vi "GetGraphVIName.vi"(8 "ErrIn (NoErr)":errorcluster caption="entrée d'erreur (pas d'erreur)", 10 "Curve Index":i32, 11 "Interface In":refnum<class "Interface.lvclass"> caption="DNL_LabVIEW Object in") -> (0 "error out":errorcluster caption="sortie d'erreur", 1 "GraphIndex":i32, 2 "GraphViNames":string[](array[string]), 3 "Interface Out":refnum<class "Interface.lvclass"> caption="DNL_LabVIEW Object out", 4 "GraphCount":i32, 6 "GraphNumbers":i32[](array[numeric]))   [LabVIEW 2019, in "Interface.lvclass"]
uses:
  Interface.lvclass
  Interface.lvclass/Interface.ctl
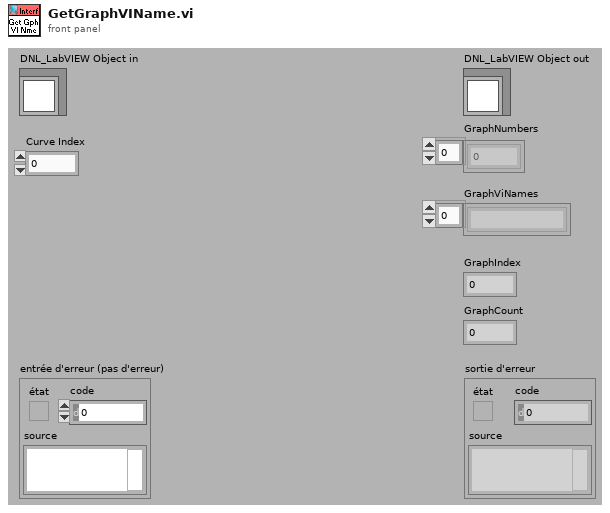
[diagram p1: front panel]
types:
  T1 = typedef "Interface.lvclass/CurveSetup.ctl" = cluster{"CurveName":string, "YParam":string, "XParam":string, "ZParam ":string, "GroupName":string, "LinWdth":u8, "PntCol":u32, "LinCol":u32, "LablFor":u8, "XScale":u32, "YScale":u32, "Interpol":u8, "DisplayName":string, "FillType":i16, "LineStyle":u8, "PntStyle":u8, "BarTyp":u8, "GraphIndex":i32, "Visible":bool, "XScaleName":string, "YScaleName":string, "XYGraph_Ref":refnum<vi>, "Data Only":bool, "DataQ Ref":refnum<queue>, "XParQ Ref":refnum<queue>, "XParamInd":i32, "ScanInd":i32, "File Path":path}
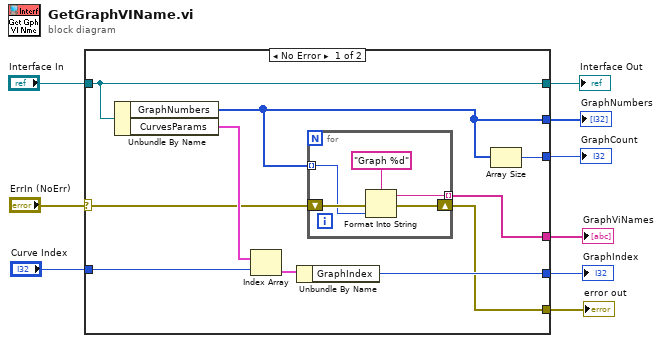
[diagram p0: block diagram]
diagram:
  n1 = case shown="No Error" "ErrIn (NoErr)" {
    selector: "ErrIn (NoErr)" -> [w12 w26]
    tunnel: [w13 w26] -> w8
    tunnel: [w19 w25] -> w6
    tunnel: "Interface In" -> [w19 w25]
    tunnel: [w11 _] -> w5
    tunnel: [w15 _] -> w4
    tunnel: "Curve Index" -> [w16 _]
    tunnel: [w14 _] -> w2
    tunnel: [w10 _] -> w1
    frame No Error {
      n2 = Unbundle By Name(w19) -> ("GraphNumbers"=w10:i32[], "CurvesParams"=w18:T1[])
      n3 = Index Array(array=w18, index=w16) -> (element=w17:T1)
      n4 = Unbundle By Name(w17) -> ("GraphIndex"=w15:i32)
      n5 = for {
        shift-right: [w22] -> w13
        shift-left: w12 -> [w23]
        tunnel: [w21] -> w11 mode=indexing
        tunnel: w10 -> [w20] mode=indexing
        n6 = Format Into String(format string="Graph %d", error in=w23, w20) -> (resulting string=w21:string, error out=w22:errorcluster)  [unwired: 1 in]
      }
      n7 = Array Size(array=w10) -> (size(s)=w14:i32)
    }
    frame Error {
    }
  }
  "error out" <- w8
  "Interface Out" <- w6
  "GraphViNames" <- w5
  "GraphIndex" <- w4
  "GraphCount" <- w2
  "GraphNumbers" <- w1
